vi "Windows Dialog Box.vi"(5 "modality (System)":enum16{"Application", "System", "Task"}(ring)=enum."System", 7 "message (\"\")":string, 8 "error in":errorcluster, 9 "icon (0:no icon)":u16(ring) items=["no icon", "STOP icon", "Question icon", "Exclamation icon", "Information icon"], 10 "buttons (0:OK)":u16(ring) items=["OK button", "OK & Cancel buttons", "Abort, Retry & Ignore buttons", "Yes, No & Cancel buttons", "Yes & No buttons", "Retry & Cancel buttons"], 11 "window title (\"\")":string) -> (0 "error out":errorcluster, 2 "button pressed":T1(ring))   [LabVIEW 2011]
doc: "This VI calls the Windows functions MessageBox and MessageBeep to display a message dialog box and, optionally, play a sound effect. These functions are in the Windows DLL called USER.EXE, which is located in the windows\\system directory. If your computer is not equipped with a sound driver, a short \"beep\" will be played through the PC's speaker.\n\nVarious combinations of dialog boxes are possible. The buttons input selects which buttons are displayed in the dialog box, the icon input determines the icon, if any, and the modality box determines whether the dialog box is system, application, or task modal.\n\nThe following dialog box button schemes are available through the \"buttons\" input:\n0: OK\n1: OK / Cancel\n2: Abort / Retry / Ignore\n3: Yes / No / Cancel\n4: Yes / No\n5: Retry / Cancel\n\nThe following icons are available through the \"icon\" input:\n0: None\n1: STOP icon\n2: Question icon\n3: Exclamation icon\n4: Information icon\n\nThe following three modalities are available:\n0: Application\n1: System\n2: Task\n\nIf sounds are enabled, the icon option determines the sound effect played, as defined in the Sounds section of Windows' Control Panel.\n\nThe DLL functions called are:\n\nint MessageBox ( hWndParent, lpText, lpCaption, wType )\nvoid MessageBeep ( wType )\n\nFunction definitions are from:\nMicrosoft Windows Programmer's Reference\nCopyright 1990 Microsoft Corporation.\n\nThe LabVIEW Technical Resource newsletter (LTR) originally distributed this VI.\nThe LTR is a quarterly publication providing technical information to LabVIEW system developers.\n\nFor subscription information, contact:\nLTR Publishing, Inc. \n6060 N. Central Expressway, Suite 502\nDallas, TX 75206\n(214) 706-0587\nFAX (214) 706-0506\nE-mail: subscribe@ltrpub.com\nwww.ltrpub.com"
uses:
  USER32.DLL
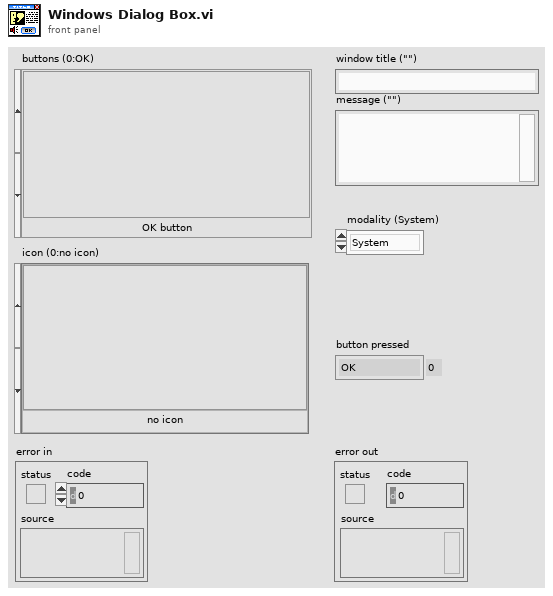
[diagram p1: front panel]
types:
  T1 = enum16{"OK", "CANCEL", "ABORT", "RETRY", "IGNORE", "YES", "NO"}
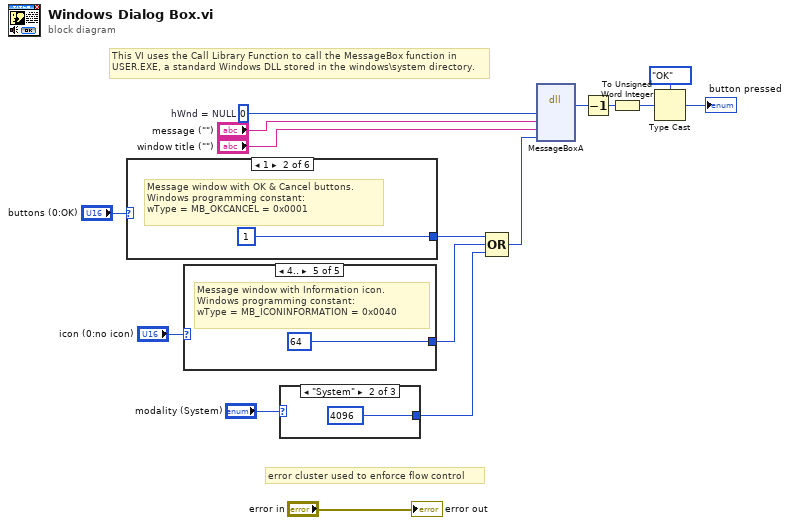
[diagram p0: block diagram]
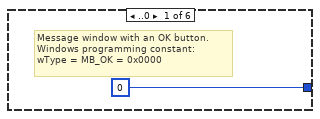
[diagram p2: hidden frame]
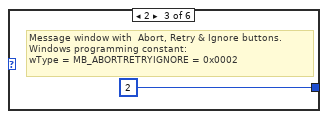
[diagram p3: hidden frame]
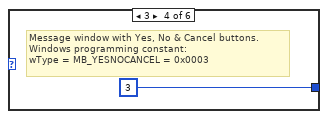
[diagram p4: hidden frame]
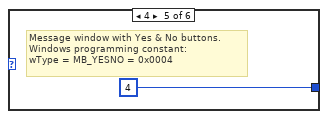
[diagram p5: hidden frame]
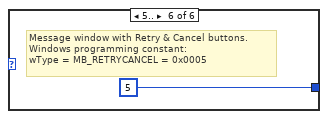
[diagram p6: hidden frame]
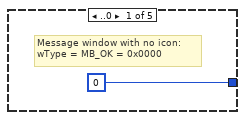
[diagram p7: hidden frame]
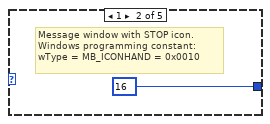
[diagram p8: hidden frame]
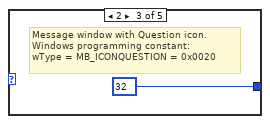
[diagram p9: hidden frame]
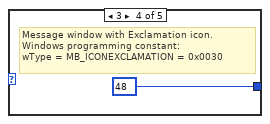
[diagram p10: hidden frame]
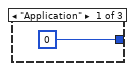
[diagram p11: hidden frame]
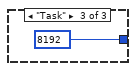
[diagram p12: hidden frame]
diagram:
  w16 = u32 0  # hWnd = NULL
  # "error cluster used to enforce flow control"
  # "This VI uses the Call Library Function to call the MessageBox function in USER.EXE, a standard Windows DLL stored in the windows\\system directory."
  n1 = case shown="1" "buttons (0:OK)" {
    tunnel: [0 1 2 3 4 5] -> w4
    frame ..0 {
      # "Message window with an OK button.\nWindows programming constant:\nwType = MB_OK = 0x0000"
    }
    frame 1 {
      # "Message window with OK & Cancel buttons.\nWindows programming constant:\nwType = MB_OKCANCEL = 0x0001"
    }
    frame 2 {
      # "Message window with  Abort, Retry & Ignore buttons.\nWindows programming constant:\nwType = MB_ABORTRETRYIGNORE = 0x0002"
    }
    frame 3 {
      # "Message window with Yes, No & Cancel buttons.\nWindows programming constant:\nwType = MB_YESNOCANCEL = 0x0003"
    }
    frame 4 {
      # "Message window with Yes & No buttons.\nWindows programming constant:\nwType = MB_YESNO = 0x0004"
    }
    frame 5.. {
      # "Message window with Retry & Cancel buttons.\nWindows programming constant:\nwType = MB_RETRYCANCEL = 0x0005"
    }
  }
  n2 = case shown="4.." "icon (0:no icon)" {
    tunnel: [0 16 32 48 64] -> w3
    frame ..0 {
      # "Message window with no icon:\nwType = MB_OK = 0x0000"
    }
    frame 1 {
      # "Message window with STOP icon.\nWindows programming constant:\nwType = MB_ICONHAND = 0x0010"
    }
    frame 2 {
      # "Message window with Question icon.\nWindows programming constant:\nwType = MB_ICONQUESTION = 0x0020"
    }
    frame 3 {
      # "Message window with Exclamation icon.\nWindows programming constant:\nwType = MB_ICONEXCLAMATION = 0x0030"
    }
    frame 4.. {
      # "Message window with Information icon.\nWindows programming constant:\nwType = MB_ICONINFORMATION = 0x0040"
    }
  }
  n3 = case shown="\"System\"" "modality (System)" {
    tunnel: [0 4096 8192] -> w2
    frame "Application" {
    }
    frame "System" {
    }
    frame "Task" {
    }
  }
  n4 = Compound Arithmetic op=OR(w4, w3, w2) -> (w1:i32)
  n5 = dll-call lib="USER32.DLL" fn="MessageBoxA" label="MessageBox"("hWndParent"=w16, "lpText"="message (\"\")", "lpCaption"="window title (\"\")", "wType"=w1) -> (w15:i32)  [unwired: 7 in, 2 out]
  n6 = Decrement(x=w15) -> (x-1=w14:i32)
  n7 = To Unsigned Word Integer(number=w14) -> (unsigned 16bit integer=w8:u16)
  n8 = Type Cast(type=T1."OK" ("button pressed"), x=w8) -> (*(type *) &x=→"button pressed":T1)
  "error out" <- "error in"
